vi "Actor Core.vi"(8 "error in":errorcluster, 11 "FE FF Frame in":refnum<class "FE FF Frame.lvclass">) -> (0 "error out":errorcluster, 3 "Actor out":refnum<class "Actor.lvclass">)   [LabVIEW 2023, in "Data Analysis.lvlib" / "FE FF Frame.lvlib" / "FE FF Frame.lvclass"]
doc: "(<B>Filename</B>: Actor Framework.lvlib:Actor.lvclass:Actor Core.vi)\n\nReceives messages to the actor, reacts to them, and initiates any error handling that may shut the actor down.\n\nDescendant classes may override this VI to append parallel tasks for the actor to complete while it handles messages. Overrides use the Call Parent Class Method node."
uses:
  FE FF Frame.lvclass
  C:/Program Files/National Instruments/LabVIEW 2023/vi.lib/ActorFramework/Actor/Actor.lvclass
  <vilib>/ActorFramework/Actor/Actor.lvclass
  FE FF Frame.lvclass/FE FF Frame.ctl
  <vilib>/ActorFramework/Actor/Actor.lvclass/Actor.ctl
  <vilib>/ActorFramework/Message Enqueuer/Message Enqueuer.lvclass/Message Enqueuer.ctl
  Subpanel-Abstract Messages/Insert SP Msg/Insert SP Msg.lvclass/Insert SP Msg.ctl
  FE FF Frame Messages/Schema Update Msg/Schema Update Msg.lvclass/Schema Update Msg.ctl
  FE FF Frame Messages/Date and Time Filter Data Msg/Date and Time Filter Data Msg.lvclass/Date and Time Filter Data Msg.ctl
  FE FF Frame Messages/Export Frame Data Msg/Export Frame Data Msg.lvclass/Export Frame Data Msg.ctl
  <vilib>/ActorFramework/Message Enqueuer/Init from Existing Queue.vi
  <vilib>/ActorFramework/Message Enqueuer/Enqueue.vi
  Subpanel-Abstract Messages/Insert SP Msg/Insert SP Msg.lvclass
  C:/Program Files/National Instruments/LabVIEW 2023/vi.lib/ActorFramework/Message/Message.lvclass
  FE FF Frame Messages/Schema Update Msg/Schema Update Msg.lvclass
  FE FF Frame Messages/Filter the Data Frame Msg/Filter the Data Frame Msg.lvclass
  FE FF Frame Messages/Date and Time Filter Data Msg/Date and Time Filter Data Msg.lvclass
  FE FF Frame Messages/Export Frame Data Msg/Export Frame Data Msg.lvclass
  <vilib>/ActorFramework/Message Priority Queue/Priority Enqueue.vi
  <vilib>/ActorFramework/Message Enqueuer/Message Enqueuer.lvclass
  Subpanel-Abstract/Subpanel-Abstract.lvclass
panel:
  in  "File Format":string(combo)="XLS"
  in  "Export Data":bool
  in  "Filter Button Time":bool
  in  "Stop Time Stamp":timestamp format="%<%x %X>T"
  in  "Start Time Stamp":timestamp format="%<%x %X>T"
  in  "Filter Button":bool
  in  "FE/FF Data":i32(listbox)=-1 caption="Data"
  in  "Stop":bool
  # "FE / FF Frame"
  # "Time Based Filter"
  # "Export Selcted Data"
  # "*All filters are applicable here"
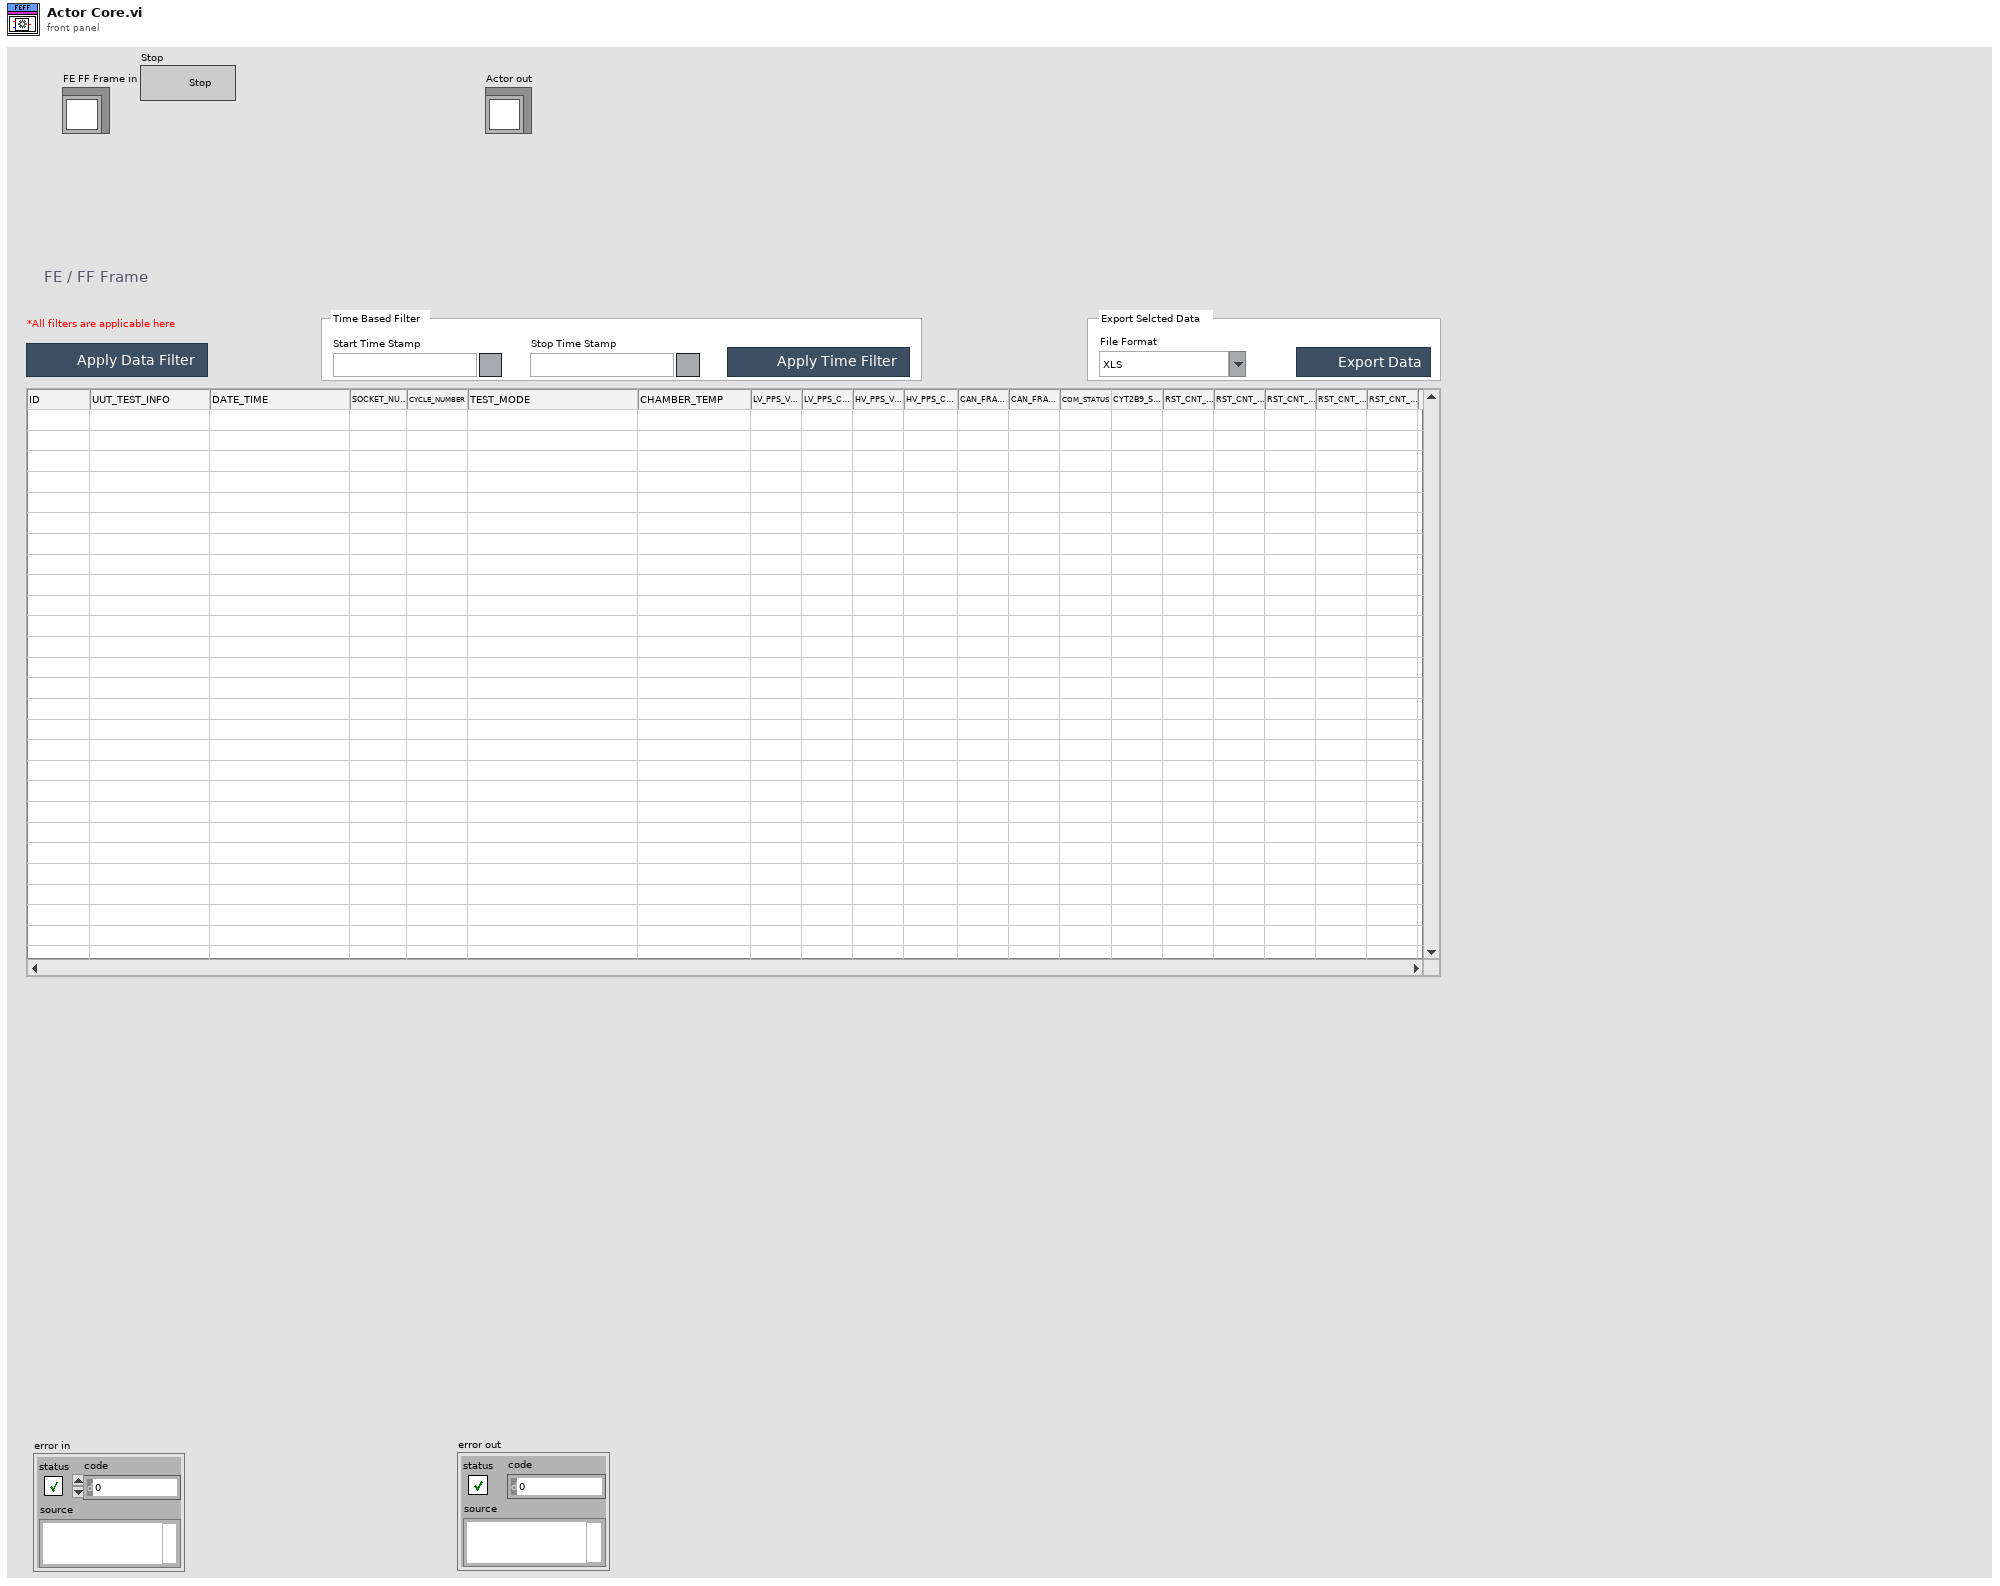
[diagram p1: front panel]
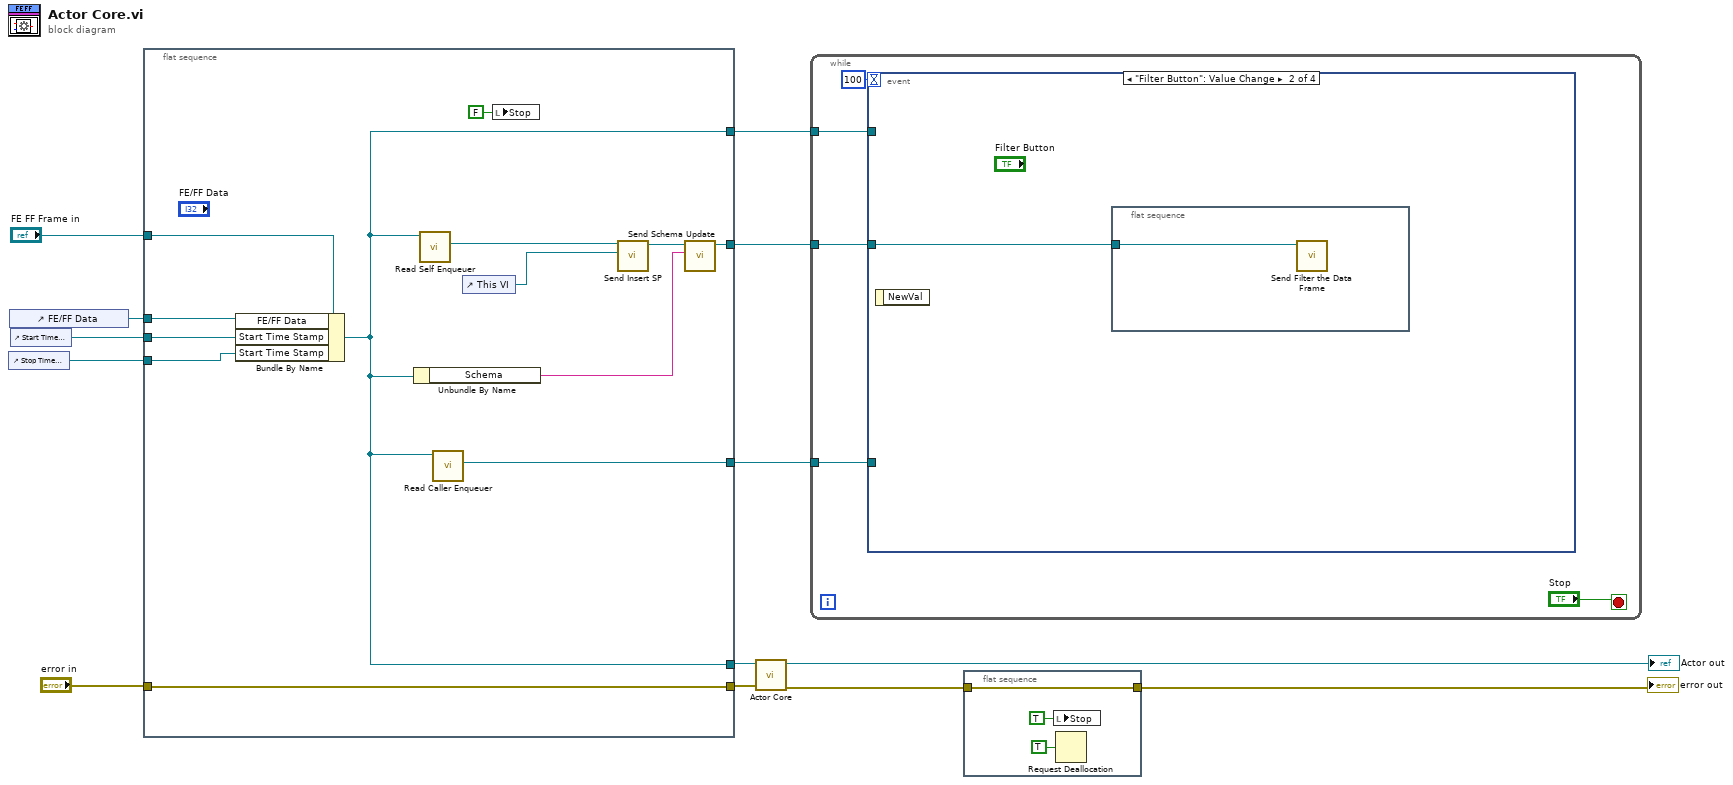
[diagram p0: block diagram]
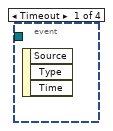
[diagram p2: hidden frame]
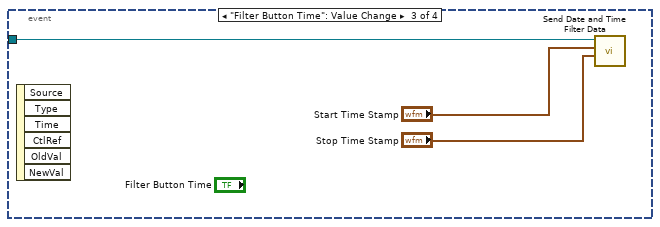
[diagram p3: hidden frame]
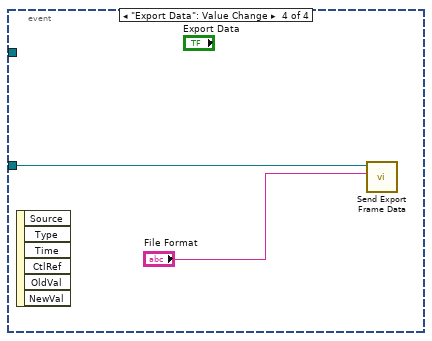
[diagram p4: hidden frame]
diagram:
  n1 = control-ref of="Stop Time Stamp"() -> (w3:refnum<vi>)
  n2 = control-ref of="FE/FF Data"() -> (w5:refnum<vi>)
  n3 = control-ref of="Start Time Stamp"() -> (w4:refnum<vi>)
  n4 = flat-sequence {
    tunnel: "error in" -> [w26]
    tunnel: [w26] -> w11
    tunnel: "FE FF Frame in" -> [w22]
    tunnel: [w15] -> w9
    tunnel: [w16] -> w6
    tunnel: w5 -> [w21]
    tunnel: w4 -> [w20]
    tunnel: w3 -> [w19]
    tunnel: [w15] -> w2
    tunnel: [w18] -> w1
    frame #0 {
      n5 = Bundle By Name(cluster=w22, "FE/FF Data"=w21, "Start Time Stamp"=w20, "Start Time Stamp"=w19) -> (w15:refnum<class "FE FF Frame.lvclass">)
      n6 = Unbundle By Name(w15) -> ("Schema"=w14:string)
      n7 = call <vilib>:"Read Self Enqueuer.vi"("Actor"=w15) -> ("Self Enqueuer"=w24:refnum<class "Message Enqueuer.lvclass">)  [unwired: 10 in]
      n8 = call <vilib>:"Read Caller Enqueuer.vi"("Actor"=w15) -> ("Caller Enqueuer"=w18:refnum<class "Message Enqueuer.lvclass">)  [unwired: 10 in]
      n9 = control-ref of="This VI"() -> (w23:refnum<vi>)
      n10 = local write "Stop"(FALSE ("Stop")) -> ()
      n11 = call "Send Insert SP.vi"("VI Ref"=w23, "Message Enqueuer"=w24) -> ("Message Enqueuer out"=w17:refnum<class "Message Enqueuer.lvclass">)  [unwired: 8 in, 1 out]
      n12 = call "Send Schema Update.vi"("Schema"=w14, "Message Enqueuer"=w17) -> ("Message Enqueuer out"=w16:refnum<class "Message Enqueuer.lvclass">)  [unwired: 8 in, 1 out]
    }
  }
  n13 = call-parent "Actor Core.vi"("error in"=w11, "Actor in"=w9) -> ("error out"=w8:errorcluster, "Actor out"=→"Actor out":refnum<class "Actor.lvclass">)  [unwired: 8 in]
  n14 = while {
    tunnel: w6 -> [w29]
    tunnel: w2 -> [w28]
    tunnel: w1 -> [w27]
    stop <- "Stop" stop-if-true
    n15 = event shown="[1] \"Filter Button\": Value Change" {
      selector: _ -> [_ _ _ _]
      dyn-events: _ -> [_ _ _ _]
      timeout: 100 -> [_ _ _ _]
      tunnel: w29 -> [_ w32 w36 w38]
      tunnel: w28 -> [_ _ _ _]
      tunnel: w27 -> [_ _ _ _]
      event Timeout {
        n16 = event-data() -> ()  [unwired: 1 in, 3 out]
      }
      event "Filter Button": Value Change {
        n17 = event-data() -> ()  [unwired: 1 in, 1 out]
        n18 = flat-sequence {
          tunnel: w32 -> [w33]
          frame #0 {
            n19 = call "Send Filter the Data Frame.vi"("Message Enqueuer"=w33) -> ()  [unwired: 9 in, 2 out]
          }
        }
      }
      event "Filter Button Time": Value Change {
        n20 = event-data() -> ()  [unwired: 1 in, 6 out]
        n21 = call "Send Date and Time Filter Data.vi"("Stop Time Stamp"="Stop Time Stamp", "Start Time Stamp"="Start Time Stamp", "Message Enqueuer"=w36) -> ()  [unwired: 7 in, 2 out]
      }
      event "Export Data": Value Change {
        n22 = event-data() -> ()  [unwired: 1 in, 6 out]
        n23 = call "Send Export Frame Data.vi"("File Format"="File Format", "Message Enqueuer"=w38) -> ()  [unwired: 8 in, 2 out]
      }
    }
  }
  n24 = flat-sequence {
    tunnel: w8 -> [w41]
    tunnel: [w41] -> w7
    frame #0 {
      n25 = local write "Stop"(TRUE ("Stop")) -> ()
      n26 = Request Deallocation(TRUE ("flag")) -> ()
    }
  }
  "error out" <- w7
